vi "Test YOLO (All Output).vi"() -> ()   [LabVIEW 2017]
doc: "Created IvanLis by LabVIEW Portal\nProfile: http://labviewportal.org/memberlist.php?mode=viewprofile&u=987\neMail: IvanLisanov@gMail.com\nTelegram: https://t.me/IvanLis"
uses:
  libonnx_wrapper/libonnx_wrapper.lvlib
  process_YOLOv8/process_YOLOv8.lvlib
  libonnx_wrapper/TypeDef/IO.ctl
  libonnx_wrapper/TypeDef/Introspection.ctl
panel:
  out "Circles":cluster{"x":sgl, "y":sgl, "r":sgl}[](array[cluster])
  out "count":i32
  out "2D Picture":picture
  out "JPG file path":path=path "/home/ivan/LabVIEWData/ONNX/LabVIEW-ONNX_Runtime/image_for_test/1_1_2r_1_1_var10.jpg"
  out "Metadata":string[][](table)
  out "Introspection Output":T1
  out "Introspection Input":T1
  out "ONNX model path":path=path "/home/ivan/LabVIEWData/ONNX/LabVIEW-ONNX_Runtime/data/coins_detection.onnx"
  out "error out":errorcluster
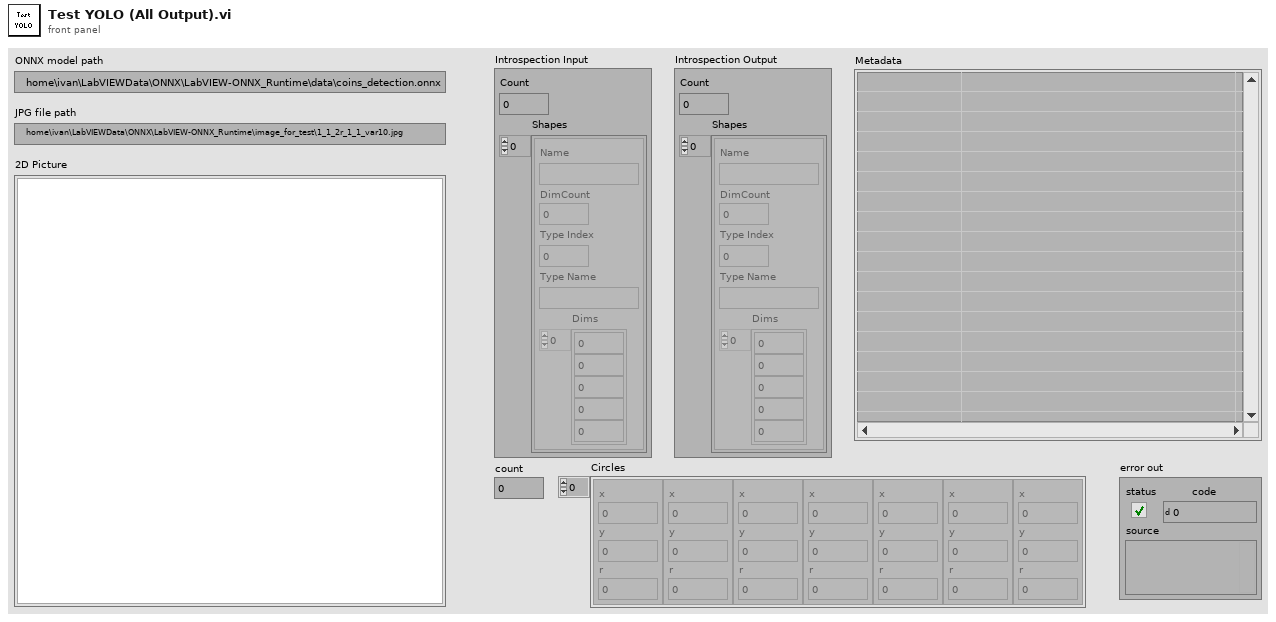
[diagram p1: front panel]
types:
  T1 = typedef "libonnx_wrapper.lvlib/Introspection.ctl" = cluster{"Count":i32, "Shapes":T2[]}
  T2 = typedef "libonnx_wrapper.lvlib/IO.ctl" = cluster{"Name":string, "DimCount":i32, "Type Index":i32, "Type Name":string, "Dims":i64[]}
  T3 = typedef "imagedata.ctl" = cluster{"image type":i32, "image depth":i32, "image":u8[], "mask":u8[], "colors":u32[], "Rectangle":cluster{"left":i16, "top":i16, "right":i16, "bottom":i16}}
  T4 = typedef "process_YOLOv8.lvlib/Circle.ctl" = cluster{"x":sgl, "y":sgl, "r":sgl}
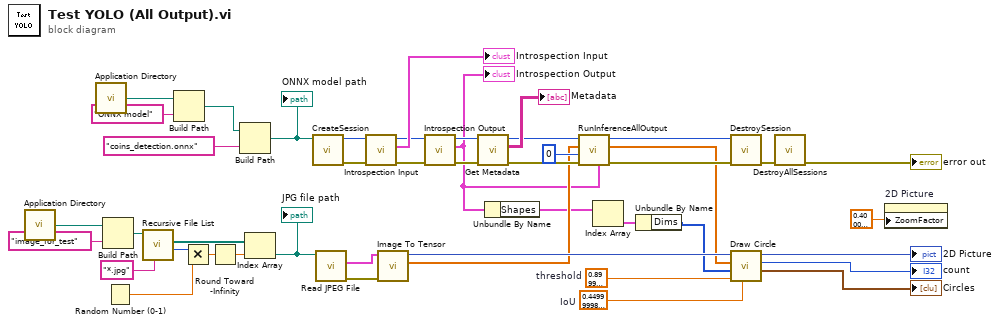
[diagram p0: block diagram]
diagram:
  w23 = sgl 0.45  # IoU
  w24 = sgl 0.9  # threshold
  n1 = call <vilib>:"Application Directory.vi"() -> ("Application Directory"=w13:path)
  n2 = call <vilib>:"Application Directory.vi"() -> ("Application Directory"=w18:path)
  n3 = Build Path(base path=w13, name or relative path="image_for_test") -> (appended path=w12:path)
  n4 = Random Number (0-1)() -> (number: 0 to 1=w10:dbl)
  n5 = call <vilib>:"Recursive File List.vi"("pattern"="*.jpg", "Folder Path"=w12) -> ("Number of Files"=w9:i32, "All Files in Dir"=w7:path[])  [unwired: 5 in, 3 out]
  n6 = Build Path(base path=w18, name or relative path="ONNX model") -> (appended path=w16:path)
  n7 = Multiply(x=w9, y=w10) -> (x*y=w8:dbl)
  n8 = Round Toward -Infinity(1:w8) -> (0:w6:dbl)
  n9 = Build Path(base path=w16, name or relative path="coins_detection.onnx") -> (appended path=w19:path)
  "ONNX model path" <- w19
  n10 = Index Array(array=w7, index=w6) -> (element=w5:path)
  "JPG file path" <- w5
  n11 = call "CreateSession.vi"("ONNX model path"=w19) -> ("error out"=w31:errorcluster, "session id out"=w32:i32)  [unwired: 9 in]
  n12 = call <vilib>:"Read JPEG File.vi"("path to JPEG file"=w5) -> ("error out"=w33:errorcluster, "image data"=w34:T3)  [unwired: 8 in, 1 out]
  n13 = call "Introspection Input.vi"("error in (no error)"=w31, "session id in"=w32) -> ("error out"=w42:errorcluster, "Introspection Input"=→"Introspection Input":T1, "session id out"=w43:i32)  [unwired: 7 in]
  n14 = call "Image To Tensor.vi"("error in (no error)"=w33, "image data"=w34) -> ("Data"=w15:sgl[], "image"=w28:picture)  [unwired: 7 in, 1 out]
  n15 = call "Introspection Output.vi"("error in (no error)"=w42, "session id in"=w43) -> ("error out"=w39:errorcluster, "Introspection Output"=w2:T1, "session id out"=w40:i32)  [unwired: 7 in]
  "Introspection Output" <- w2
  n16 = call "Get Metadata.vi"("error in (no error)"=w39, "session id in"=w40) -> ("error out"=w36:errorcluster, "Metadata"=→"Metadata":string[][], "session id out"=w37:i32)  [unwired: 7 in]
  n17 = Unbundle By Name(w2) -> ("Shapes"=w4:T2[])
  n18 = call "RunInferenceAllOutput.vi"("Introspection Output"=w2, "error in (no error)"=w36, "inputIndex"=0, "inputBuffer"=w15, "session id in"=w37) -> ("error out"=w30:errorcluster, "outputBuffer"=w25:sgl[], "session id out"=w29:i32)  [unwired: 4 in]
  n19 = Index Array(array=w4) -> (element=w3:T2)  [unwired: 1 in]
  n20 = Unbundle By Name(w3) -> ("Dims"=w1:i64[])
  n21 = call "DestroySession.vi"("error in (no error)"=w30, "session id in"=w29) -> ("error out"=w45:errorcluster)  [unwired: 8 in, 1 out]
  n22 = call "Draw Circle.vi"("IoU"=w23, "threshold"=w24, "dim"=w1, "data"=w25, "image in"=w28) -> ("Circles"=→"Circles":T4[], "count"=→"count":i32, "image out"=→"2D Picture":picture)  [unwired: 4 in]
  n23 = call "DestroyAllSessions.vi"("error in (no error)"=w45) -> ("error out"=→"error out":errorcluster)  [unwired: 10 in]
  n24 = property on="2D Picture" class="Pict"("ZoomFactor"=sgl 0.4 ("Zoom Factor")) -> ()  [unwired: 2 in, 2 out]
